vi "Write commandStart.vi"(8 "error in (no error)":errorcluster, 10 "commandStart":dbl, 11 "SettingUpState in":refnum<class "SettingUpState.lvclass">) -> (0 "error out":errorcluster, 3 "SettingUpState out":refnum<class "SettingUpState.lvclass">)   [LabVIEW 2020, in "SettingUpState.lvclass"]
uses:
  SettingUpState.lvclass
  SettingUpState.lvclass/SettingUpState.ctl
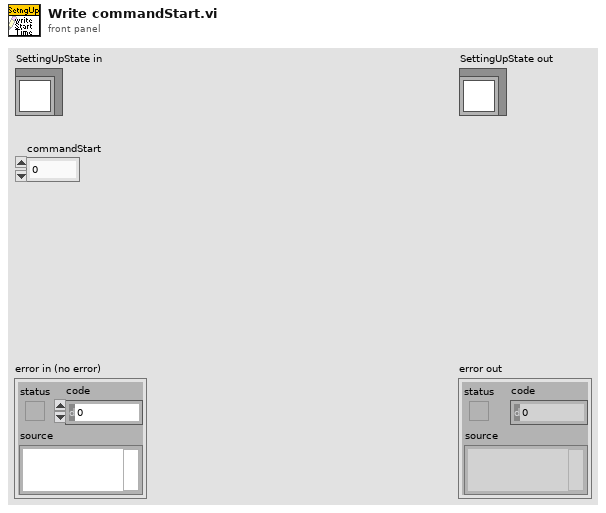
[diagram p1: front panel]
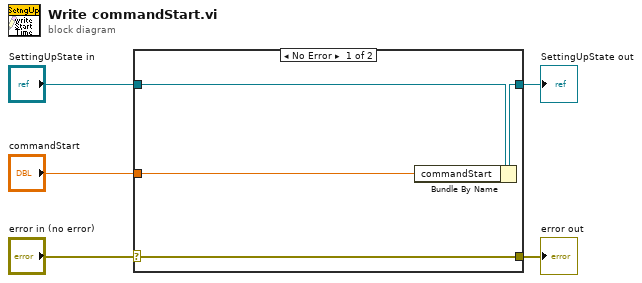
[diagram p0: block diagram]
diagram:
  n1 = case shown="No Error" "error in (no error)" {
    selector: "error in (no error)" -> [w9 w10]
    tunnel: [w9 w10] -> w4
    tunnel: [w7 w11] -> w2
    tunnel: "SettingUpState in" -> [w8 w11]
    tunnel: "commandStart" -> [w6 _]
    frame No Error {
      n2 = Bundle By Name(cluster=w8, "commandStart"=w6) -> (w7:refnum<class "SettingUpState.lvclass">)
    }
    frame Error {
    }
  }
  "error out" <- w4
  "SettingUpState out" <- w2
